vi "Generate Fade.vi"(10 "Fade in? (True)":bool=TRUE, 11 "Original Sound":refnum<class "Sound.lvclass">=refnum) -> (3 "Fade":refnum<class "Fade.lvclass">)   [LabVIEW 2010, in "Fade.lvclass"]
uses:
  Fade.lvclass
  Sound Modification/Sound Modification.lvclass
  Sound/Sound.lvclass
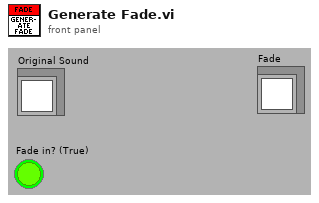
[diagram p1: front panel]
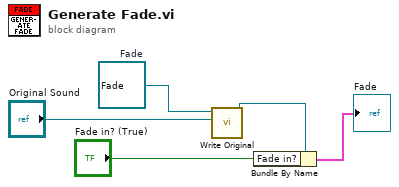
[diagram p0: block diagram]
diagram:
  w5 = refnum<class "Fade.lvclass"> refnum  # Fade
  n1 = call "Write Original.vi"("Sound.lvclass"="Original Sound", "Sound Modification in"=w5) -> ("Sound Modification out"=w1:refnum<class "Sound Modification.lvclass">)  [unwired: 9 in]
  n2 = Bundle By Name(cluster=w1, "Fade in?"="Fade in? (True)") -> (→"Fade":cluster{})
